vi "Engine - Generic - HPCR_Plot.vi"() -> ()   [LabVIEW 2015, in "ECS-Host.lvlib"]
uses:
  ECS-Host.lvlib
panel:
  out "RailPStp":sgl caption="[]" min=0 max=0.2 step=0.001 format="%#.3f"
  out "IMVDutyCyc_Des":sgl=0.7671859 caption="[]"
  out "HPVDutyCyc_Des":sgl=0.7671859 caption="[]"
  out "RailP":sgl caption="[]" min=0 max=0.2 step=0.001 format="%#.3f"
  out "_RailP Chart":T1(graph)
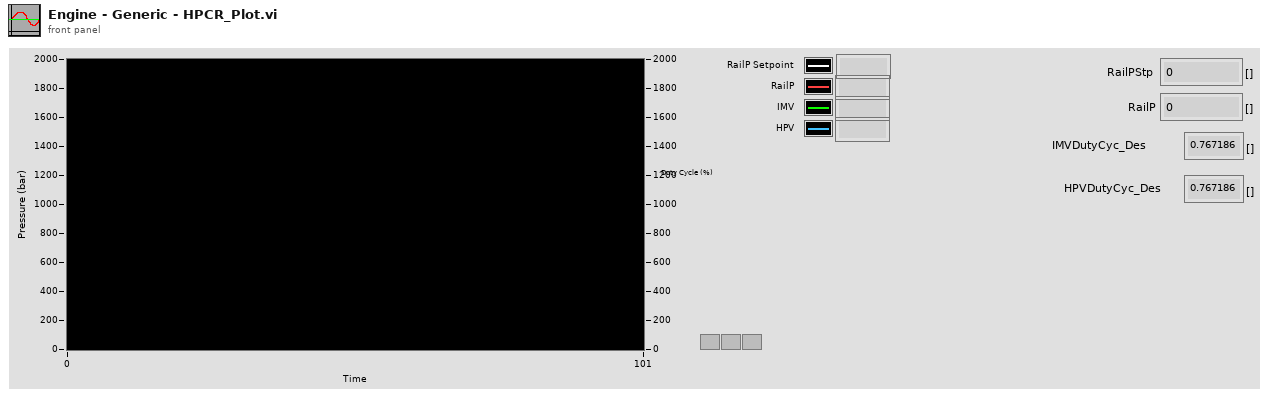
[diagram p1: front panel]
types:
  T1 = cluster{"RailP_Setpoint":sgl, "RailP":sgl, "IMV_DC":sgl, "HPV_DC":sgl}
  T2 = cluster{"RailPStp":sgl, "RailP":sgl, "IMVDutyCyc_Des":sgl, "HPVDutyCyc_Des":sgl}
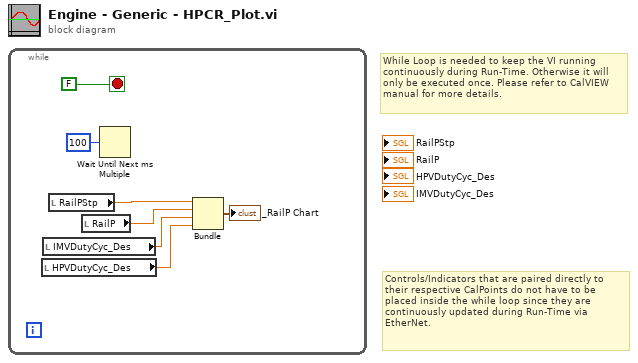
[diagram p0: block diagram]
diagram:
  # "Controls/Indicators that are paired directly to their respective CalPoints do not have to be placed inside the while loop since they are continuously updated during Run-Time via EtherNet."
  # "While Loop is needed to keep the VI running\ncontinuously during Run-Time. Otherwise it will only be executed once. Please refer to CalVIEW manual for more details."
  n1 = while {
    stop <- FALSE stop-if-true
    n2 = local read "HPVDutyCyc_Des"() -> (w3:sgl)
    n3 = local read "IMVDutyCyc_Des"() -> (w2:sgl)
    n4 = local read "RailPStp"() -> (w1:sgl)
    n5 = local read "RailP"() -> (w4:sgl)
    n6 = Wait Until Next ms Multiple(millisecond multiple=u32 100) -> ()  [unwired: 1 out]
    n7 = Bundle("RailPStp"=w1, "RailP"=w4, "IMVDutyCyc_Des"=w2, "HPVDutyCyc_Des"=w3) -> (→"_RailP Chart":T2)  [unwired: 1 out]
  }
